vi "CheckModules.vi"(8 "Your Suppose":i32[][](array[numeric]), 11 "Last Draw":i64[](array[numeric])) -> (0 "Matches":i32[][](array[numeric]), 1 "Sum":i32, 2 "Matches 2":i32[](array[numeric]))   [LabVIEW 2023]
uses:
  <vilib>/Utility/file.llb/Write Delimited Spreadsheet (I64).vi
panel:
  out "Залози":i32[][](array[numeric])
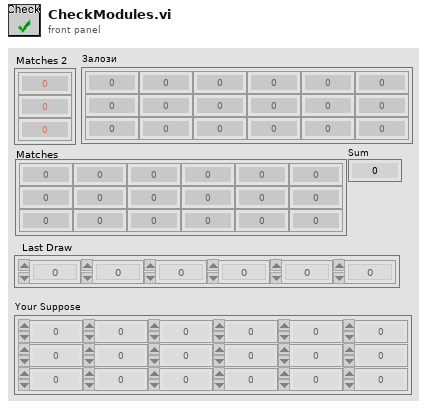
[diagram p1: front panel]
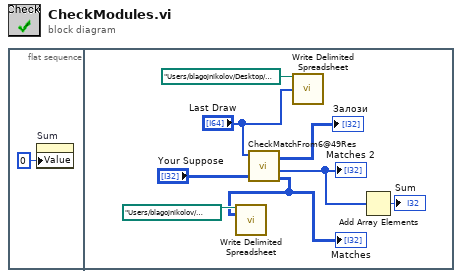
[diagram p0: block diagram]
diagram:
  n1 = flat-sequence {
    frame #0 {
      n2 = property on="Sum" class="DigNum (strict)"("Value"=0 ("sum")) -> ()  [unwired: 2 in, 2 out]
    }
    frame #1 {
      n3 = call "CheckMatchFrom6@49Res.vi"("Твоето предположение"="Your Suppose", "Последен тираж"="Last Draw") -> (0:w6:i64[][], "Съвпадения"=w3:i32[], "Залози"=→"Залози":i32[][])  [unwired: 6 in, 1 out]
      "Matches 2" <- w3
      "Matches" <- w6
      n4 = call-poly <vilib>:"Write Delimited Spreadsheet.vi"("file path (dialog if empty)"=path "/Users/blagojnikolov/Desktop/@tmp/matches1.txt", "2D data"=w6) -> ()  [unwired: 12 in, 2 out]
      n5 = call-poly <vilib>:"Write Delimited Spreadsheet.vi"("file path (dialog if empty)"=path "/Users/blagojnikolov/Desktop/@tmp/officialResults.txt", "1D data"="Last Draw") -> ()  [unwired: 12 in, 2 out]
      n6 = Add Array Elements(numeric array=w3) -> (sum=→"Sum":i32)
    }
  }
